vi "串口初始化.vi"(11 "VISA引用句柄输入":refnum<visa-resource-name>) -> (0 "错误输出":errorcluster caption="error out", 3 "VISA引用句柄输出":refnum<visa-resource-name>)   [LabVIEW 2014]
uses:
  <vilib>/Instr/_visa.llb/VISA Configure Serial Port (Instr).vi
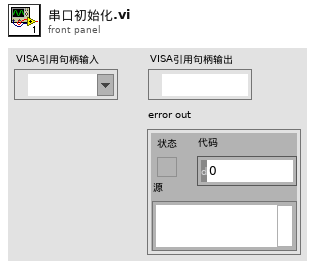
[diagram p1: front panel]
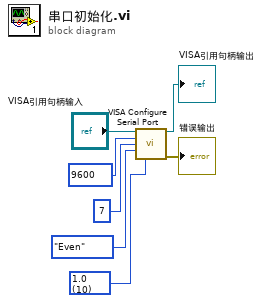
[diagram p0: block diagram]
diagram:
  w7 = u16 10 items=["1.0"=10, "1.5"=15, "2.0"=20] ("停止位")
  n1 = call-poly "VISA Configure Serial Port"("VISA resource name"="VISA引用句柄输入", "baud rate (9600)"=u32 9600 ("波特率"), "data bits (8)"=u16 7 ("数据位"), "parity (0:none)"=enum16{"None", "Odd", "Even", "Mark", "Space"}."Even" ("校验位"), "stop bits (10: 1 bit)"=w7) -> ("VISA resource name out"=→"VISA引用句柄输出":refnum<visa-resource-name>, "error out"=→"错误输出":errorcluster)  [unwired: 9 in]
